vi "Tank to Arcade Drive.vi"(2 "Left":dbl, 3 "Right":dbl) -> (0 "Y":dbl, 1 "X":dbl)   [LabVIEW 2016]
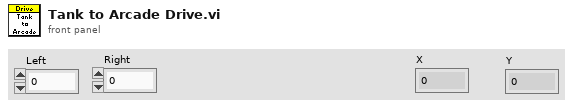
[diagram p1: front panel]
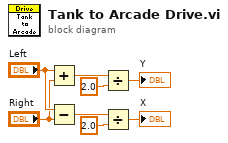
[diagram p0: block diagram]
diagram:
  n1 = Add(x="Left", y="Right") -> (x+y=w5:dbl)
  n2 = Subtract(x="Left", y="Right") -> (x-y=w8:dbl)
  n3 = Divide(x=w5, y=2.0) -> (x/y=→"Y":dbl)
  n4 = Divide(x=w8, y=2.0) -> (x/y=→"X":dbl)
